vi "Read Working Values.vi"(0 "VISA resource name":refnum<visa-resource-name>, 1 "Unit Address (1)":u8=1 min=1 max=254, 11 "error in (no error)":errorcluster) -> (4 "VISA resource name out":refnum<visa-resource-name>, 6 "Working Setpoint (0)":sgl, 10 "Working Output (0)":sgl format="%#_4g", 15 "error out":errorcluster)   [LabVIEW 2010, in "Eurotherm 32xx Series.lvlib"]
doc: "This VI returns Working Values."
uses:
  <instrlib>/Eurotherm 32xx Series/Eurotherm 32xx Series.lvlib
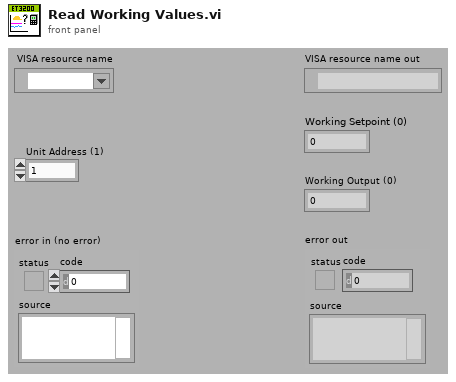
[diagram p1: front panel]
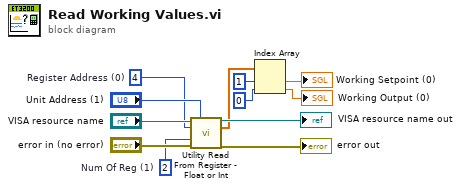
[diagram p0: block diagram]
diagram:
  w4 = u16 4  # Register Address (0)
  w7 = u16 2  # Num Of Reg (1)
  n1 = call <instrlib>:"Utility Read From Register - Float or Int.vi"("VISA resource name"="VISA resource name", "Unit Address (1)"="Unit Address (1)", "Register Address (0)"=w4, "Num Of Reg (1)"=w7, "error in (no error)"="error in (no error)") -> ("VISA resource name out"=→"VISA resource name out":refnum<visa-resource-name>, "Data"=w6:sgl[], "error out"=→"error out":errorcluster)  [unwired: 8 in]
  n2 = Index Array(array=w6, index #1=1 ("index"), index #2=0 ("index")) -> (element #1=→"Working Setpoint (0)":sgl, element #2=→"Working Output (0)":sgl)
